vi "Adjust Decoration.vi"(6 "Control Ref Queue":T4, 8 "error in (no error)":errorcluster, 10 "Matrix Representation Array In":T1, 11 "2D Plotmatrix.lvclass in":refnum<class "XY Plot Matrix.lvclass">) -> (0 "error out":errorcluster, 2 "Matrix Representation Array Out":T1, 3 "2D Plotmatrix.lvclass out":refnum<class "XY Plot Matrix.lvclass">)   [LabVIEW 2017, in "XY Plot Matrix.lvclass"]
uses:
  <vilib>/Math Plots/2D Math Plots/XY Plot Matrix/XY Plot Matrix/XY Plot Matrix.lvclass
  <vilib>/Math Plots/2D Math Plots/2D Plot/Action String/XYPlotMatrix Ctrl Act Queue.ctl
  <vilib>/Math Plots/2D Math Plots/2D Plot/Action String/XYPlotMatrix Ctrl Act Cluster.ctl
  <vilib>/Math Plots/2D Math Plots/2D Plot/Action String/2DMathPlot State Class.ctl
  <vilib>/Math Plots/2D Math Plots/XY Plot Matrix/XY Plot Matrix/Typedef/Mulitmatrix Representation.ctl
  <vilib>/Math Plots/2D Math Plots/XY Plot Matrix/XY Plot Matrix/Typedef/Matrix Representation.ctl
  <vilib>/Math Plots/2D Math Plots/2D Plot/2D Plot/Typedef/Range Cluster.ctl
  <vilib>/Utility/miscctls.llb/LVPositionTypeDef.ctl
  <vilib>/Math Plots/2D Math Plots/2D Plot/2D Plot/2D Plot.lvclass
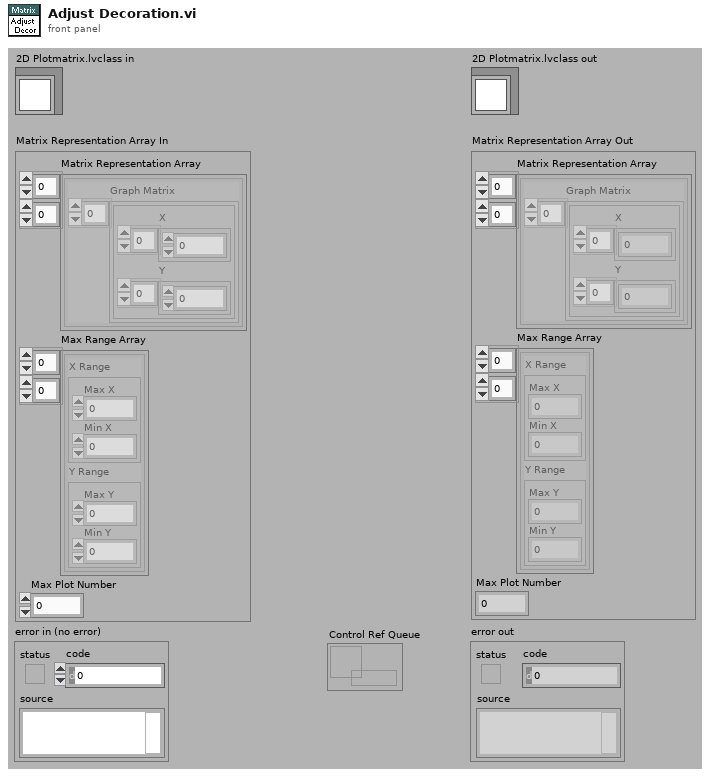
[diagram p1: front panel]
types:
  T1 = typedef "XY Plot Matrix.lvclass/Mulitmatrix Representation.ctl" = cluster{"Matrix Representation Array":T2[][], "Max Range Array":T3[][], "Max Plot Number":i32}
  T2 = typedef "XY Plot Matrix.lvclass/Matrix Representation.ctl" = cluster{"Graph Matrix":cluster{"X":dbl[], "Y":dbl[]}[]}
  T3 = typedef "2D Plot.lvclass/Range Cluster.ctl" = cluster{"X Range":cluster{"Max X":dbl, "Min X":dbl}, "Y Range":cluster{"Max Y":dbl, "Min Y":dbl}}
  T4 = typedef "XYPlotMatrix Ctrl Act Queue.ctl" = refnum<queue>
  T5 = typedef "LVPositionTypeDef.ctl" = cluster{"Left":i32, "Top":i32}
  T6 = typedef "XYPlotMatrix Ctrl Act Cluster.ctl" = cluster{"Facade VI":refnum<vi>, "XControl":refnum<vi>, "Sub Panel":refnum<vi>, "Sub VI":refnum<vi>, "Export Image":refnum<vi>, "Display State Change Class":T7}
  T7 = typedef "2DMathPlot State Class.ctl" = enum16{"Update All (Undo)", "Update General", "Update Appearance", "Update Format", "Update Scale", "Update Marker", "Update Cursor", "None"}
  T8 = typedef "LVBoundsTypeDef.ctl" = cluster{"Width":u32, "Height":u32}
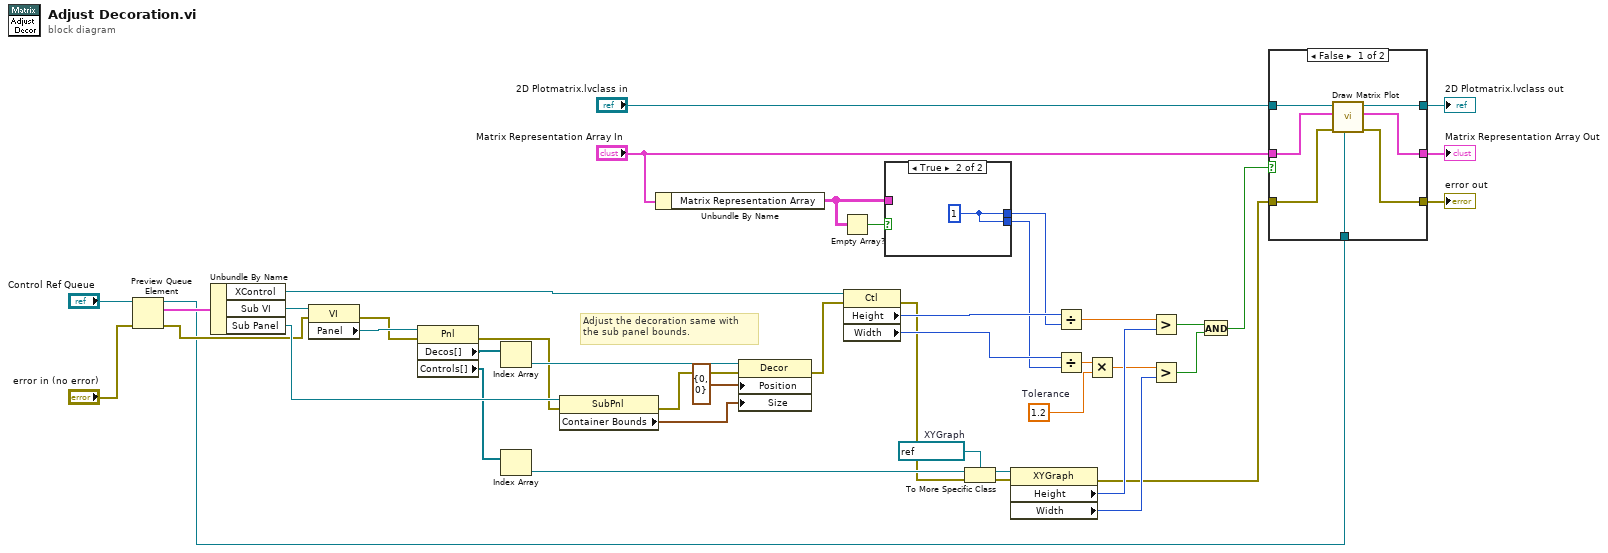
[diagram p0: block diagram]
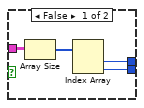
[diagram p2: hidden frame]
diagram:
  w6 = 1.2  # Tolerance
  w28 = refnum<vi> refnum  # XYGraph
  # "Adjust the decoration same with \nthe sub panel bounds."
  n1 = Preview Queue Element(queue="Control Ref Queue", error in (no error)="error in (no error)") -> (queue out=w11:T4, element=w43:T6, error out=w34:errorcluster)  [unwired: 2 out]
  n2 = Unbundle By Name(w43) -> ("XControl"=w26:refnum<vi>, "Sub VI"=w41:refnum<vi>, "Sub Panel"=w38:refnum<vi>)
  n3 = property class="VI"(reference=w41, error in=w34) -> (error out=w33:errorcluster, "Panel"=w40:refnum<vi>)  [unwired: 1 out]
  n4 = property class="Pnl"(reference=w40, error in=w33) -> (error out=w35:errorcluster, "Decos[]"=w39:refnum<vi>[], "Controls[]"=w30:refnum<vi>[])  [unwired: 1 out]
  n5 = Index Array(array=w39) -> (element=w37:refnum<vi>)  [unwired: 1 in]
  n6 = Index Array(array=w30) -> (element=w29:refnum<vi>)  [unwired: 1 in]
  n7 = property class="SubPnl"(reference=w38, error in=w35) -> (error out=w36:errorcluster, "Container Bounds"=w31:T8)  [unwired: 1 out]
  n8 = Unbundle By Name("Matrix Representation Array In") -> ("Matrix Representation Array"=w4:T2[][])
  n9 = property class="Decor"(reference=w37, error in=w36, "Position"=T5 {"Left"=0, "Top"=0}, "Size"=w31) -> (error out=w8:errorcluster)  [unwired: 1 out]
  n10 = Empty Array?(array=w4) -> (empty?=w3:bool)
  n11 = property class="Ctl"(reference=w26, error in=w8) -> (error out=w2:errorcluster, "Height"=w25:u32, "Width"=w23:u32)  [unwired: 1 out]
  n12 = case shown="True" w3 {
    tunnel: [w47 w49] -> w24
    tunnel: [w46 w49] -> w22
    tunnel: w4 -> [w45 _]
    frame False {
      n13 = Array Size(array=w45) -> (size(s)=w48:i32[])
      n14 = Index Array(array=w48) -> (element #1=w47:i32, element #2=w46:i32)  [unwired: 2 in]
    }
    frame True {
      w49 = 1
    }
  }
  n15 = To More Specific Class(target class=w28, reference=w29, error in=w2) -> (specific class reference=w27:refnum<vi>, error out=w1:errorcluster)
  n16 = property class="XYGraph"(reference=w27, error in=w1) -> (error out=w9:errorcluster, "Height"=w21:u32, "Width"=w19:u32)  [unwired: 1 out]
  n17 = Divide(x=w25, y=w24) -> (x/y=w5:dbl)
  n18 = Divide(x=w23, y=w22) -> (x/y=w20:dbl)
  n19 = Multiply(x=w20, y=w6) -> (x*y=w7:dbl)
  n20 = Greater?(x=w5, y=w21) -> (0:w18:bool)
  n21 = Greater?(x=w7, y=w19) -> (0:w17:bool)
  n22 = And(x=w18, y=w17) -> (x .and. y?=w16:bool)
  n23 = case shown="False" w16 {
    tunnel: "2D Plotmatrix.lvclass in" -> [w56 w58]
    tunnel: [w55 w58] -> w14
    tunnel: "Matrix Representation Array In" -> [w54 w59]
    tunnel: [w53 w59] -> w12
    tunnel: w11 -> [w52 _]
    tunnel: [w51 w57] -> w10
    tunnel: w9 -> [w50 w57]
    frame False {
      n24 = call <vilib>:"Draw Matrix Plot.vi"("Control Ref Queue"=w52, "error in (no error)"=w50, "Matrix Representation Array In"=w54, "2D Plotmatrix.lvclass in"=w56) -> ("error out"=w51:errorcluster, "Matrix Representation Array Out"=w53:T1, "2D Plotmatrix.lvclass out"=w55:refnum<class "XY Plot Matrix.lvclass">)  [unwired: 5 out]
    }
    frame True {
      # "The XY graph is in \ncorrect order. Pass"
    }
  }
  "error out" <- w10
  "2D Plotmatrix.lvclass out" <- w14
  "Matrix Representation Array Out" <- w12
